vi "Configure Measurement Limits.vi"(5 "Fail Counter Auto Clear Mode (1: On)":u16(ring)=1 items=["Off", "On", "Once"], 6 "Maximum Power (90.0 dBm)":dbl=90.0 format="%#.6g", 7 "Minimum Power (-90.0 dBm)":dbl=-90.0 format="%#.6g", 8 "error in (no error)":errorcluster, 9 "Enable Limits (F: Disable)":bool, 10 "Measurement Number (1: Measurement 1)":u16(ring)=1 items=["Measurement 1"=1, "Measurement 2"=2, "Measurement 3"=3, "Measurement 4"=4], 11 "VISA resource name":refnum<visa-resource-name>) -> (0 "error out":errorcluster, 3 "VISA resource name out":refnum<visa-resource-name>)   [LabVIEW 2011, in "Agilent N432A.lvlib"]
doc: "Enables/disables the test limits for the specified window and sets both the upper and lower level limits. It also sets the Fail Counter Auto Clear Mode."
uses:
  <instrlib>/Agilent N432A/Agilent N432A.lvlib
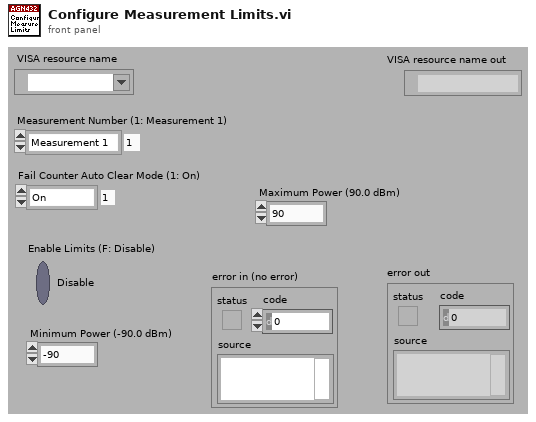
[diagram p1: front panel]
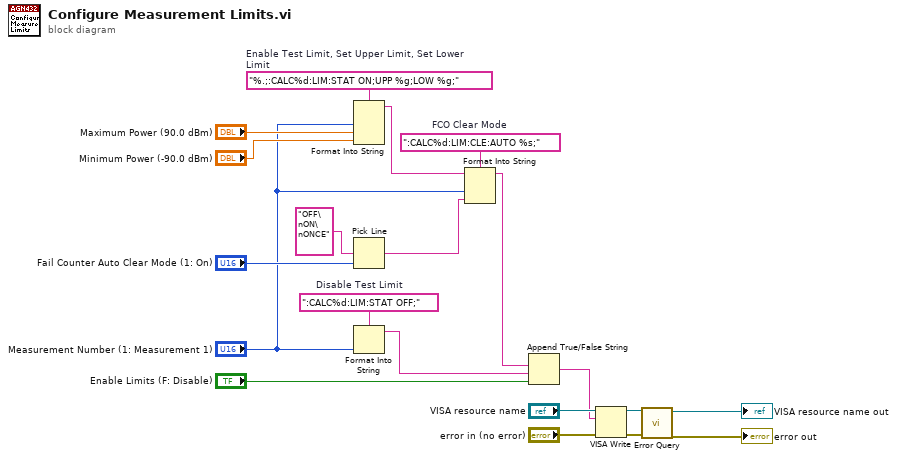
[diagram p0: block diagram]
diagram:
  w7 = ":CALC%d:LIM:CLE:AUTO %s;"  # FCO Clear Mode
  w8 = "%.;:CALC%d:LIM:STAT ON;UPP %g;LOW %g;"  # Enable Test Limit, Set Upper Limit, Set Lower Limit
  w11 = ":CALC%d:LIM:STAT OFF;"  # Disable Test Limit
  n1 = Format Into String(format string=w8, "Measurement Number (1: Measurement 1)", "Maximum Power (90.0 dBm)", "Minimum Power (-90.0 dBm)") -> (resulting string=w6:string)  [unwired: 2 in, 1 out]
  n2 = Pick Line(multi-line string="OFF\nON\nONCE", line index="Fail Counter Auto Clear Mode (1: On)") -> (output string=w5:string)  [unwired: 1 in]
  n3 = Format Into String(format string=w11, "Measurement Number (1: Measurement 1)") -> (resulting string=w10:string)  [unwired: 2 in, 1 out]
  n4 = Format Into String(format string=w7, initial string=w6, "Measurement Number (1: Measurement 1)", w5) -> (resulting string=w3:string)  [unwired: 1 in, 1 out]
  n5 = Append True/False String(1:"Enable Limits (F: Disable)", 2:w10, 3:w3) -> (0:w12:string)  [unwired: 1 in]
  n6 = VISA Write(VISA resource name="VISA resource name", write buffer=w12, error in (no error)="error in (no error)") -> (VISA resource name out=w2:refnum<visa-resource-name>, error out=w1:errorcluster)  [unwired: 1 out]
  n7 = call <instrlib>:"Error Query.vi"("error in (no error)"=w1, "VISA resource name"=w2) -> ("error out"=→"error out":errorcluster, "VISA resource name out"=→"VISA resource name out":refnum<visa-resource-name>)  [unwired: 6 in, 2 out]
